vi "ma_Design FIR Coeff.vi"(8 "error in":errorcluster, 9 "Optional FIR Filter Specifications":T3={"PB Gain"=3.0, "SB Gain"=60.0, "Scale"=TRUE, "Window"=enum."Flat Top"} {"SB Gain" format="%0.2f"; "PB Gain" format="%0.2f"}, 10 "FIR Filter Specifications":T2={"Topology"=enum."Off", "Type"=enum."Bandstop", "#Taps"=1500, "Lower PB"=1500.0, "Upper PB"=1500.0, "Lower SB"=0.0, "Upper SB"=0.0} {"Lower SB" format="%0.2p"; "Upper SB" format="%0.2p"; "Lower PB" format="%0.2p"; "Upper PB" format="%0.2p"}, 11 "Sampling Frequency":dbl format="%0.2f") -> (0 "error out":errorcluster, 2 "Forward Coefficients":dbl[](array[numeric]) format="%0.2f", 3 "Filter Information":T1 {"phase H(w)"."df" format="%0.2f"; "phase H(w)"."f0" format="%0.2f"; "phase H(w)"."Phase H(w)" format="%0.2f"; "magnitude H(w)"."df" format="%0.2f"; "magnitude H(w)"."f0" format="%0.2f"; "magnitude H(w)"."Mag H(w)" format="%0.2f"})   [LabVIEW 2020, in "NI_MAPro.lvlib"]
uses:
  NI_MAPro.lvlib
  NI_AALBase.lvlib
  NI_MABase.lvlib
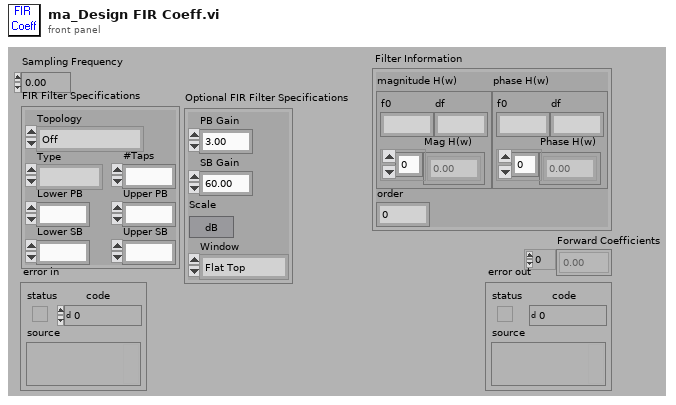
[diagram p1: front panel]
types:
  T1 = cluster{"magnitude H(w)":cluster{"f0":dbl, "df":dbl, "Mag H(w)":dbl[]}, "phase H(w)":cluster{"f0":dbl, "df":dbl, "Phase H(w)":dbl[]}, "order":i32}
  T2 = cluster{"Topology":enum16{"Off", "FIR by Specification", "Equi-ripple FIR", "Windowed FIR"}, "Type":enum16{"Lowpass", "Highpass", "Bandpass", "Bandstop"}, "#Taps":i32, "Lower PB":dbl, "Upper PB":dbl, "Lower SB":dbl, "Upper SB":dbl}
  T3 = cluster{"PB Gain":dbl, "SB Gain":dbl, "Scale":bool, "Window":enum16{"None", "Hanning", "Hamming", "Triangular", "Blackman", "Exact Blackman", "Blackman-Harris", "Kaiser-Bessel", "Flat Top"}}
  T4 = enum16{"Off", "FIR by Specification", "Equi-ripple FIR", "Windowed FIR"}
  T5 = cluster{"Lower PB":dbl, "Upper PB":dbl, "Lower SB":dbl, "Upper SB":dbl, "PB Gain":dbl, "SB Gain":dbl, "Scale":bool}
  T6 = enum16{"Lowpass", "Highpass", "Bandpass", "Bandstop"}
  T7 = enum16{"None", "Hanning", "Hamming", "Triangular", "Blackman", "Exact Blackman", "Blackman-Harris", "Kaiser-Bessel", "Flat Top"}
  T8 = cluster{"amplitude":dbl, "lower freq":dbl, "higher freq":dbl, "ripple weight":dbl}[]
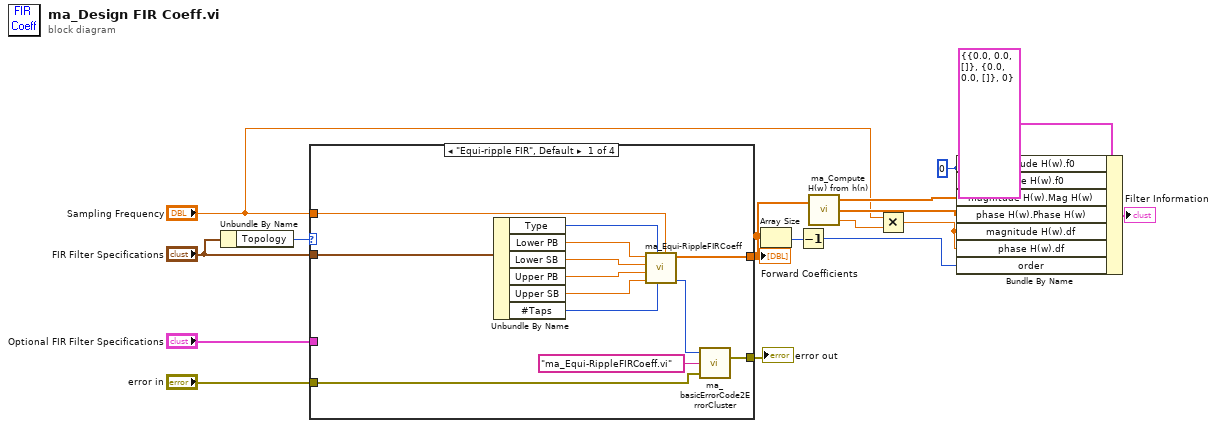
[diagram p0: block diagram]
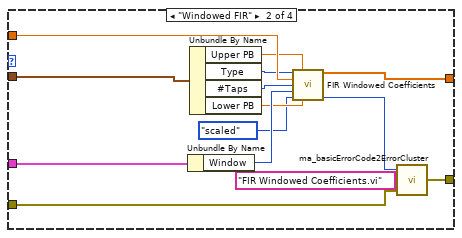
[diagram p2: hidden frame]
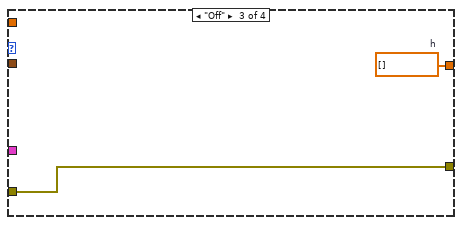
[diagram p3: hidden frame]
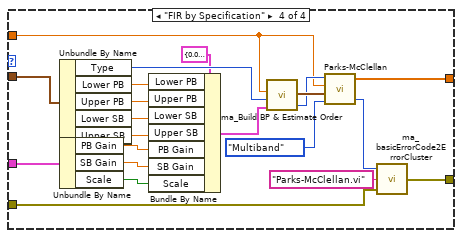
[diagram p4: hidden frame]
diagram:
  w5 = 0
  n1 = Unbundle By Name("FIR Filter Specifications") -> ("Topology"=w12:T4)
  n2 = case shown="\"Equi-ripple FIR\", Default" w12 {
    tunnel: "Sampling Frequency" -> [w22 w42 _ w57]
    tunnel: [w20 w36 w44 w66] -> w14
    tunnel: [w29 w43 w45 w64] -> w11
    tunnel: "Optional FIR Filter Specifications" -> [_ w41 _ w62]
    tunnel: "FIR Filter Specifications" -> [w28 w39 _ w61]
    tunnel: "error in" -> [w19 w35 w44 w60]
    frame "Equi-ripple FIR", Default {
      n3 = Unbundle By Name(w28) -> ("Type"=w23:T6, "Lower PB"=w24:dbl, "Lower SB"=w25:dbl, "Upper PB"=w26:dbl, "Upper SB"=w27:dbl, "#Taps"=w21:i32)
      n4 = call "ma_Equi-RippleFIRCoeff.vi"("sampling freq: fs"=w22, "# of taps"=w21, "Filter type"=w23, "higher stop freq"=w27, "higher pass freq"=w26, "lower stop freq"=w25, "lower pass freq"=w24) -> ("error"=w18:i32, "FIR Coefficients"=w29:dbl[])  [unwired: 2 in, 1 out]
      n5 = call "ma_basicErrorCode2ErrorCluster.vi"("error in (no error)"=w19, "subVI name"="ma_Equi-RippleFIRCoeff.vi", "Error Code"=w18) -> ("error out"=w20:errorcluster)
    }
    frame "Windowed FIR" {
      n6 = Unbundle By Name(w41) -> ("Window"=w40:T7)
      n7 = Unbundle By Name(w39) -> ("Upper PB"=w31:dbl, "Type"=w38:T6, "#Taps"=w37:i32, "Lower PB"=w32:dbl)
      n8 = call "FIR Windowed Coefficients.vi"("filter type"=w38, "high cutoff freq: fh"=w31, "sampling freq: fs"=w42, "taps"=w37, "window"=w40, "option"=enum32{"not scaled", "scaled"}."scaled", "low cutoff freq: fl"=w32) -> ("FIR Windowed Coefficients"=w43:dbl[], "error"=w34:i32)  [unwired: 7 in]
      n9 = call "ma_basicErrorCode2ErrorCluster.vi"("error in (no error)"=w35, "subVI name"="FIR Windowed Coefficients.vi", "Error Code"=w34) -> ("error out"=w36:errorcluster)
    }
    frame "Off" {
      w45 = dbl[] []  # h
    }
    frame "FIR by Specification" {
      n10 = Unbundle By Name(w61) -> ("Type"=w56:T6, "Lower PB"=w49:dbl, "Upper PB"=w50:dbl, "Lower SB"=w51:dbl, "Upper SB"=w52:dbl)
      n11 = Unbundle By Name(w62) -> ("PB Gain"=w53:dbl, "SB Gain"=w54:dbl, "Scale"=w55:bool)
      n12 = Bundle By Name(cluster=T5 {"Lower PB"=0.0, "Upper PB"=0.0, "Lower SB"=0.0, "Upper SB"=0.0, "PB Gain"=0.0, "SB Gain"=0.0, "Scale"=FALSE} ("Desired Filter Specifications"), "Lower PB"=w49, "Upper PB"=w50, "Lower SB"=w51, "Upper SB"=w52, "PB Gain"=w53, "SB Gain"=w54, "Scale"=w55) -> (w47:T5)
      n13 = call "ma_Build BP & Estimate Order.vi"("Desired Filter Specifications"=w47, "Filter type"=w56, "Sampling Frequency"=w57) -> ("filter order"=w58:i32, "Band Parameters"=w59:T8)  [unwired: 2 in]
      n14 = call "Parks-McClellan.vi"("filter type"=enum32{"Multiband", "Differentiator", "Hilbert"}."Multiband", "Band Parameters"=w59, "sampling freq: fs"=w57, "# of taps"=w58) -> ("error"=w65:i32, "h"=w64:dbl[])  [unwired: 1 out]
      n15 = call "ma_basicErrorCode2ErrorCluster.vi"("error in (no error)"=w60, "subVI name"="Parks-McClellan.vi", "Error Code"=w65) -> ("error out"=w66:errorcluster)
    }
  }
  "Forward Coefficients" <- w11
  "error out" <- w14
  n16 = Array Size(array=w11) -> (size(s)=w10:i32)
  n17 = Decrement(x=w10) -> (x-1=w7:i32)
  n18 = call "ma_Compute H(w) from h(n).vi"("h"=w11) -> ("Mag H(w)"=w9:dbl[], "Phase H(w)"=w8:dbl[], "df"=w4:dbl)  [unwired: 1 in]
  n19 = Multiply(x="Sampling Frequency", y=w4) -> (x*y=w3:dbl)
  n20 = Bundle By Name(cluster=T1 {"magnitude H(w)"={"f0"=0.0, "df"=0.0, "Mag H(w)"=[]}, "phase H(w)"={"f0"=0.0, "df"=0.0, "Phase H(w)"=[]}, "order"=0} ("Filter Information"), "magnitude H(w).f0"=w5, "phase H(w).f0"=w5, "magnitude H(w).Mag H(w)"=w9, "phase H(w).Phase H(w)"=w8, "magnitude H(w).df"=w3, "phase H(w).df"=w3, "order"=w7) -> (→"Filter Information":T1)
